vi "util_queue_status.vi"(7 "references":T1, 8 "error in (no error)":errorcluster) -> (0 "error out":errorcluster)   [LabVIEW 2015, in "repub-dvr_nre.lvlib"]
uses:
  repub-dvr_nre.lvlib
  public/_controls/references.ctl
  _controls/input.ctl
  _controls/input_command.ctl
  _controls/output.ctl
  _controls/data.ctl
  public/_controls/configuration.ctl
  lv-recipe-machine/private/_controls/recipe_data.ctl
  lv-recipe-machine/public/_controls/mode.ctl
  lv-recipe-machine/public/_controls/manual_state.ctl
  lv-recipe-machine/public/_controls/automatic_state.ctl
  <userlib>/antonio-alexander/lv-waitgroup/public/_controls/api_waitgroup.ctl
  lv-recipe-machine/public/_controls/transition.ctl
  public/_controls/change.ctl
  public/_controls/status.ctl
  lv-recipe-machine/lv-recipe-machine.lvlib
  <userlib>/antonio-alexander/lv-waitgroup/lv-waitgroup.lvlib
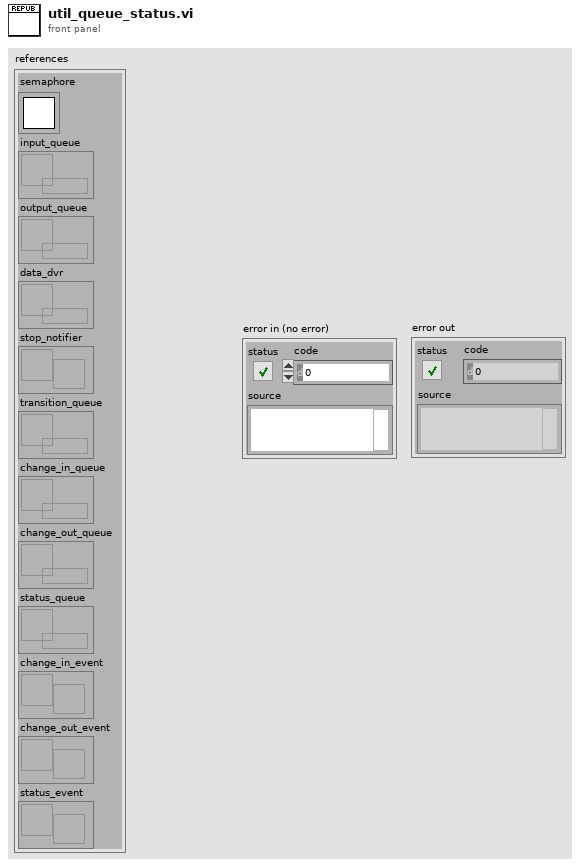
[diagram p1: front panel]
types:
  T1 = typedef "repub-dvr_nre.lvlib/references.ctl" = cluster{"semaphore":T2, "input_queue":refnum<queue>, "output_queue":refnum<queue>, "data_dvr":refnum<data-value>, "stop_notifier":refnum<notifier>, "transition_queue":refnum<queue>, "change_in_queue":refnum<queue>, "change_out_queue":refnum<queue>, "status_queue":refnum<queue>, "change_in_event":refnum<user-event>, "change_out_event":refnum<user-event>, "status_event":refnum<user-event>}
  T2 = typedef "Semaphore RefNum" = refnum<k1>
  T3 = typedef "repub-dvr_nre.lvlib/status.ctl" = cluster{"mode":T4, "manual_state":T5, "automatic_state":T6, "step":string}
  T4 = typedef "lv-recipe-machine.lvlib/mode.ctl" = enum16{"<mode>", "manual", "automatic", "<null>"}
  T5 = typedef "lv-recipe-machine.lvlib/manual_state.ctl" = enum16{"<manual_state>", "failed", "action", "running", "idle", "<null>"}
  T6 = typedef "lv-recipe-machine.lvlib/automatic_state.ctl" = enum16{"<automatic_state>", "failed", "idle", "running", "paused", "transition", "stopped", "<null>"}
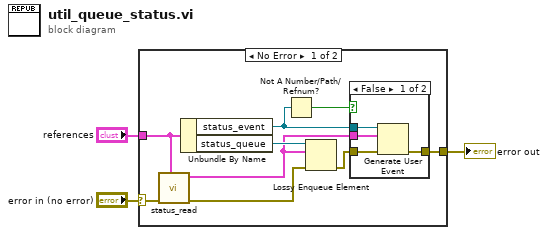
[diagram p0: block diagram]
diagram:
  n1 = case shown="No Error" "error in (no error)" {
    selector: "error in (no error)" -> [w8 w18]
    tunnel: "references" -> [w12 _]
    tunnel: [w5 w18] -> w1
    frame No Error {
      n2 = call "status_read.vi"("references"=w12, "error in (no error)"=w8) -> ("error out"=w9:errorcluster, "status"=w10:T3)  [unwired: 8 in]
      n3 = Unbundle By Name(w12) -> ("status_event"=w6:refnum<user-event>, "status_queue"=w11:refnum<queue>)
      n4 = Not A Number/Path/Refnum?(number/path/refnum=w6) -> (NaN/Path/Refnum?=w4:bool)
      n5 = Lossy Enqueue Element(queue=w11, element=w10, error in (no error)=w9) -> (error out=w7:errorcluster)  [unwired: 3 out]
      n6 = case shown="False" w4 {
        tunnel: w10 -> [w16 _]
        tunnel: w7 -> [w15 w17]
        tunnel: w6 -> [w14 _]
        tunnel: [w13 w17] -> w5
        frame False {
          n7 = Generate User Event(user event=w14, event data cluster=w16, error in=w15) -> (error out=w13:errorcluster)  [unwired: 1 in, 1 out]
        }
        frame True {
        }
      }
    }
    frame Error {
    }
  }
  "error out" <- w1
